vi "Teleop.vi"(10 "Match Info":T1={"Autonomous Elapsed Seconds"=0.0, "TeleOp Elapsed Seconds"=0.0, "Disabled Elapsed Seconds"=0.0, "Visited Autonomous"=FALSE, "Visited TeleOp"=FALSE, "Visited Disabled"=FALSE, "Autonomous Settings"={"Autonomous Style"=enum."Independent", "VI Refnum"=refnum}}, 11 "Call Context":T2) -> ()   [LabVIEW 2011]
doc: "This VI is called for each TeleOp packet received from the DS where the robot is not disabled. It is often used to read from the joysticks and update I/O or to update setpoints for timed control loops. It should complete and return within 20 milliseconds or it may miss DS packets."
uses:
  <vilib>/Rock Robotics/WPI/DriverStation/WPI_DriverStationDerivedRobotMode.ctl
  <vilib>/Rock Robotics/WPI/DriverStation/WPI_DriverStationMatch Info.ctl
  Robot Global Data.vi
panel:
  out "Shift Control":dbl=2.0 format="%.2f"
  in  "Left High":dbl=0.2
  in  "Right High":dbl=0.8
  in  "Left Mid":dbl=0.25
  in  "Right Mid":dbl=0.7
  in  "Shift Input 2":dbl
  in  "Left Low":dbl=0.8
  in  "Right Low":dbl=0.4
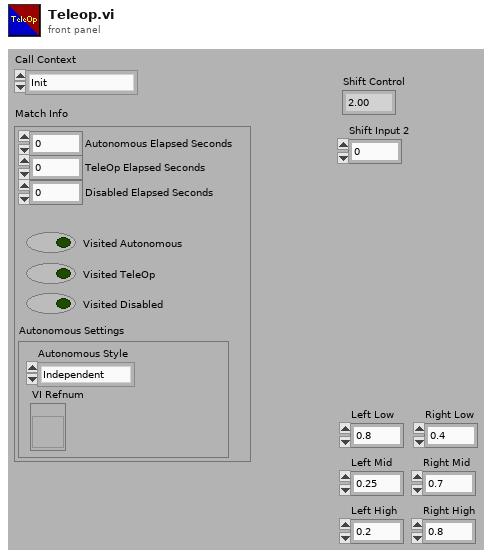
[diagram p1: front panel]
types:
  T1 = typedef "WPI_DriverStationMatch Info.ctl" = cluster{"Autonomous Elapsed Seconds":dbl, "TeleOp Elapsed Seconds":dbl, "Disabled Elapsed Seconds":dbl, "Visited Autonomous":bool, "Visited TeleOp":bool, "Visited Disabled":bool, "Autonomous Settings":cluster{"Autonomous Style":enum16{"Iterative", "Independent"}, "VI Refnum":refnum<vi>}}
  T2 = typedef "WPI_DriverStationDerivedRobotMode.ctl" = enum16{"Init", "Execute", "Stop"}
  T3 = typedef "WPI_MotorControlDeviceRef.ctl" = cluster{"DeviceStatus":errorcluster, "Type":enum16{"PWM", "CAN"}, "PWM":cluster{"Digital Module":T4, "PWM Channel":T5, "DeadBand":T6}, "CAN":cluster{"Device Number":u8, "Control Mode":T7, "Semaphore":T8, "Max Vout":dbl}, "Invert":bool, "TransformRef":T9, "InvTransformRef":T9}
  T4 = typedef "FPGA_TypedefDigitalModule.ctl" = enum16{"Digital Module 1", "Digital Module 2"}
  T5 = typedef "FPGA_DIOPWMChannel.ctl" = enum8{"PWM 1", "PWM 2", "PWM 3", "PWM 4", "PWM 5", "PWM 6", "PWM 7", "PWM 8", "PWM 9", "PWM 10", "Invalid"}
  T6 = typedef "WPI_PWMDeadband.ctl" = cluster{"Name":string, "maxPositivePwm":i32, "minPositivePwm":i32, "centerPwm":i32, "maxNegativePwm":i32, "minNegativePwm":i32, "angularRange":u16}
  T7 = typedef "WPI_CANJaguar_ControlMode.ctl" = enum8{"Percent VBus", "Current", "Speed", "Position", "Voltage"}
  T8 = typedef "Semaphore RefNum" = refnum<k1>
  T9 = typedef "WPI_PWMTransform_ConPane.ctl" = refnum<vi>
  T10 = typedef "WPI_ServoDeviceRef.ctl" = cluster{"DeviceStatus":errorcluster, "Digital Module":T4, "PWM Channel":T5, "DeadBand":T6}
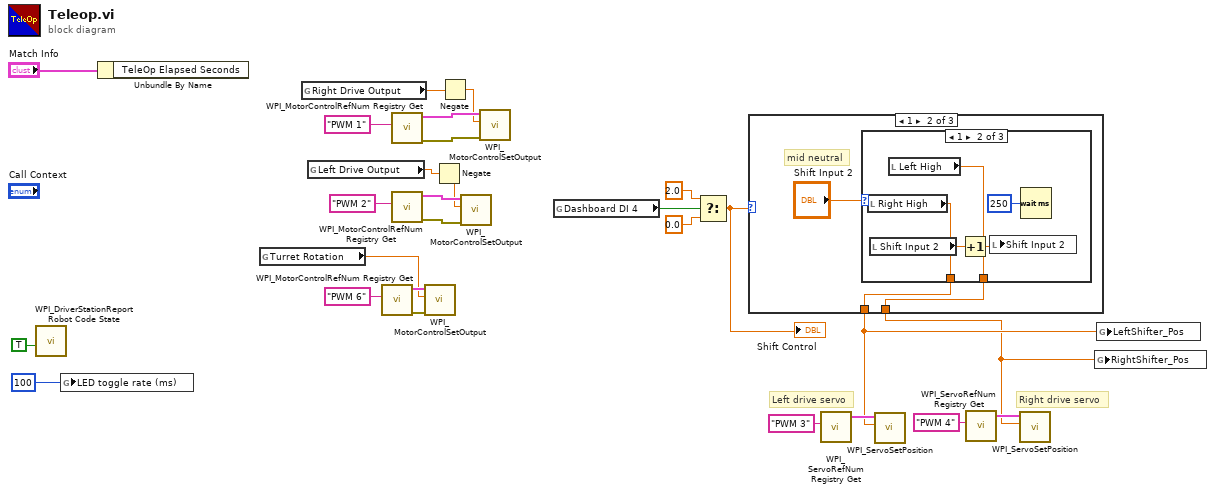
[diagram p0: block diagram]
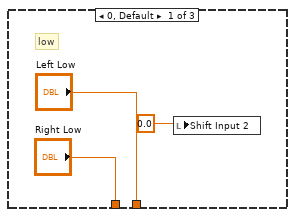
[diagram p2: hidden frame]
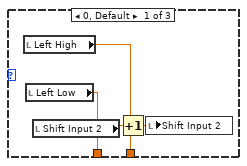
[diagram p3: hidden frame]
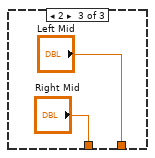
[diagram p4: hidden frame]
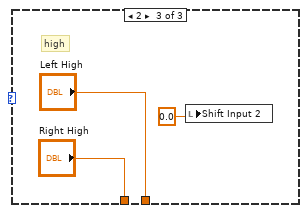
[diagram p5: hidden frame]
diagram:
  # "Right drive servo"
  # "Left drive servo"
  n1 = call <vilib>:"WPI_DriverStationReport Robot Code State.vi"("TeleOp"=TRUE ("Autonomous")) -> ()  [unwired: 10 in, 1 out]
  n2 = global write "Robot Global Data.vi" "LED toggle rate (ms)"(u32 100 ("LED ms toggle rate")) -> ()
  n3 = Unbundle By Name("Match Info") -> ()  [unwired: 1 out]
  n4 = global read "Robot Global Data.vi" "Turret Rotation"() -> (w1:dbl)
  n5 = global read "Robot Global Data.vi" "Right Drive Output"() -> (w8:dbl)
  n6 = global read "Robot Global Data.vi" "Left Drive Output"() -> (w5:dbl)
  n7 = call <vilib>:"WPI_MotorControlRefNum Registry Get.vi"("refnum name"="PWM 6") -> ("error out"=w4:errorcluster, "MotorControlDevRef"=w3:T3)  [unwired: 9 in]
  n8 = call <vilib>:"WPI_MotorControlRefNum Registry Get.vi"("refnum name"="PWM 1") -> ("error out"=w21:errorcluster, "MotorControlDevRef"=w22:T3)  [unwired: 9 in]
  n9 = call <vilib>:"WPI_MotorControlRefNum Registry Get.vi"("refnum name"="PWM 2") -> ("error out"=w19:errorcluster, "MotorControlDevRef"=w20:T3)  [unwired: 9 in]
  n10 = call <vilib>:"WPI_MotorControlSetOutput.vi"("error in (no error)"=w4, "Output"=w1, "MotorControlDevRef"=w3) -> ()  [unwired: 7 in, 2 out]
  n11 = Negate(x=w5) -> (-x=w6:dbl)
  n12 = Negate(x=w8) -> (-x=w7:dbl)
  n13 = call <vilib>:"WPI_MotorControlSetOutput.vi"("error in (no error)"=w19, "Output"=w6, "MotorControlDevRef"=w20) -> ()  [unwired: 7 in, 2 out]
  n14 = call <vilib>:"WPI_MotorControlSetOutput.vi"("error in (no error)"=w21, "Output"=w7, "MotorControlDevRef"=w22) -> ()  [unwired: 7 in, 2 out]
  n15 = global read "Robot Global Data.vi" "Dashboard DI 4"() -> (w11:bool)
  n16 = Select(t=2.0, s=w11, f=0.0) -> (s? t:f=w13:dbl)
  "Shift Control" <- w13
  n17 = case shown="1" w13 {
    tunnel: ["Left Low" w32 "Left High"] -> w9
    tunnel: ["Right Low" w31 "Right High"] -> w10
    frame 0, Default {
      # "low"
      n18 = local write "Shift Input 2"(0.0 ("Input 2")) -> ()
    }
    frame 1 {
      # "mid neutral"
      n19 = case shown="1" "Shift Input 2" {
        tunnel: [w37 w38 "Left Mid"] -> w32
        tunnel: [w36 w39 "Right Mid"] -> w31
        frame 0, Default {
          n20 = local read "Left High"() -> (w37:dbl)
          n21 = local read "Left Low"() -> (w36:dbl)
          n22 = local read "Shift Input 2"() -> (w35:dbl)
          n23 = Increment(x=w35) -> (x+1=w34:dbl)
          n24 = local write "Shift Input 2"(w34) -> ()
        }
        frame 1 {
          n25 = local read "Right High"() -> (w39:dbl)
          n26 = local read "Shift Input 2"() -> (w41:dbl)
          n27 = local read "Left High"() -> (w38:dbl)
          n28 = Increment(x=w41) -> (x+1=w40:dbl)
          n29 = local write "Shift Input 2"(w40) -> ()
          n30 = Wait (ms)(milliseconds to wait=u32 250) -> ()  [unwired: 1 out]
        }
        frame 2 {
        }
      }
    }
    frame 2 {
      # "high"
      n31 = local write "Shift Input 2"(0.0 ("Input 2")) -> ()
    }
  }
  n32 = call <vilib>:"WPI_ServoRefNum Registry Get.vi"("refnum name"="PWM 3") -> ("ServoDeviceRef"=w18:T10)  [unwired: 1 in, 9 out]
  n33 = call <vilib>:"WPI_ServoSetPosition.vi"("Position"=w10, "ServoDeviceRef"=w18) -> ()  [unwired: 1 in, 9 out]
  n34 = call <vilib>:"WPI_ServoRefNum Registry Get.vi"("refnum name"="PWM 4") -> ("ServoDeviceRef"=w14:T10)  [unwired: 1 in, 9 out]
  n35 = call <vilib>:"WPI_ServoSetPosition.vi"("Position"=w9, "ServoDeviceRef"=w14) -> ()  [unwired: 1 in, 9 out]
  n36 = global write "Robot Global Data.vi" "RightShifter_Pos"(w9) -> ()
  n37 = global write "Robot Global Data.vi" "LeftShifter_Pos"(w10) -> ()
